vi "ABB Report HV Test.vi"(10 "Report in":string) -> (2 "Report out":string)   [LabVIEW 2017]
uses:
  ABB global.vi
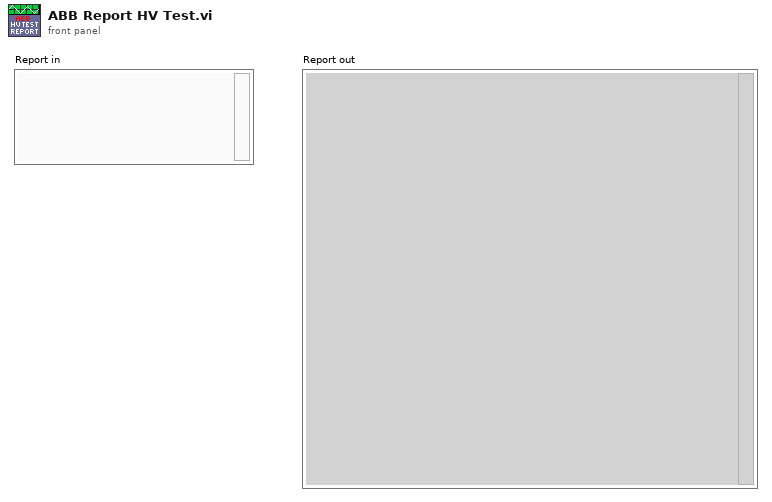
[diagram p1: front panel]
types:
  T1 = cluster{"Prior to test":dbl, "Prior v":dbl, "Prior temp":dbl, "After test":dbl, "after v":dbl, "After temp":dbl, "Test Voltage (kV)":dbl, "Test Time (min)":dbl}
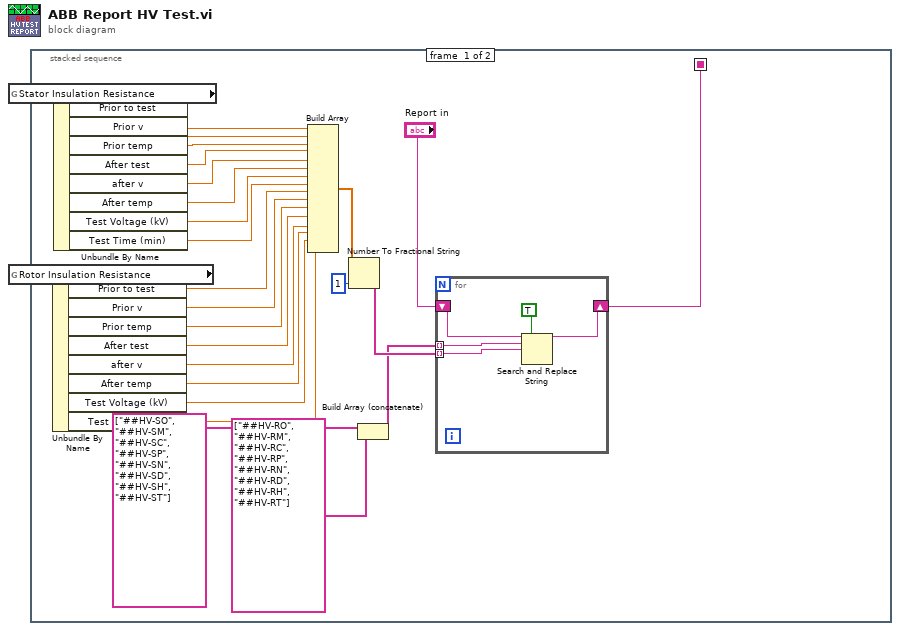
[diagram p0: block diagram]
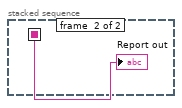
[diagram p2: hidden frame]
diagram:
  n1 = stacked-sequence {
    seq-local: [w24 _] -> [_ w32]
    frame #0 {
      n2 = global read "ABB global.vi" "Stator Insulation Resistance"() -> (w26:T1)
      n3 = global read "ABB global.vi" "Rotor Insulation Resistance"() -> (w11:T1)
      n4 = Unbundle By Name(w11) -> ("Prior to test"=w10:dbl, "Prior v"=w9:dbl, "Prior temp"=w8:dbl, "After test"=w7:dbl, "after v"=w6:dbl, "After temp"=w5:dbl, "Test Voltage (kV)"=w4:dbl, "Test Time (min)"=w3:dbl)
      n5 = Unbundle By Name(w26) -> ("Prior to test"=w19:dbl, "Prior v"=w18:dbl, "Prior temp"=w17:dbl, "After test"=w16:dbl, "after v"=w15:dbl, "After temp"=w14:dbl, "Test Voltage (kV)"=w13:dbl, "Test Time (min)"=w12:dbl)
      n6 = Build Array(w19, w18, w17, w16, w15, w14, w13, w12, w10, w9, w8, w7, w6, w5, w4, w3) -> (w22:dbl[])
      n7 = Number To Fractional String(number=w22, precision (6)=i16 1) -> (F-format string=w20:string[])  [unwired: 2 in]
      n8 = Build Array (concatenate)(string[] ["##HV-SO", "##HV-SM", "##HV-SC", "##HV-SP", "##HV-SN", "##HV-SD", "##HV-SH", "##HV-ST"], string[] ["##HV-RO", "##HV-RM", "##HV-RC", "##HV-RP", "##HV-RN", "##HV-RD", "##HV-RH", "##HV-RT"]) -> (w2:string[])
      n9 = for {
        shift-right: [w31] -> w24
        shift-left: "Report in" -> [w30]
        tunnel: w2 -> [w28] mode=indexing
        tunnel: w20 -> [w27] mode=indexing
        n10 = Search and Replace String(replace all?=TRUE ("replace all? (F)"), input string=w30, search string=w28, replace string=w27) -> (result string=w31:string)  [unwired: 4 in, 3 out]
      }
    }
    frame #1 {
      "Report out" <- w32
    }
  }
